vi "ILABW_RemoteCommandMgr.vi"(0 "action":string, 1 "data":string, 4 "errorIn":errorcluster) -> (5 "response":string, 7 "errorOut":string)   [LabVIEW 2012]
panel:
  in  "vi":string
  out "Control":bool
  out "Connection Status":string
  in  "Case Constant\n(See Context Help)":bool=TRUE
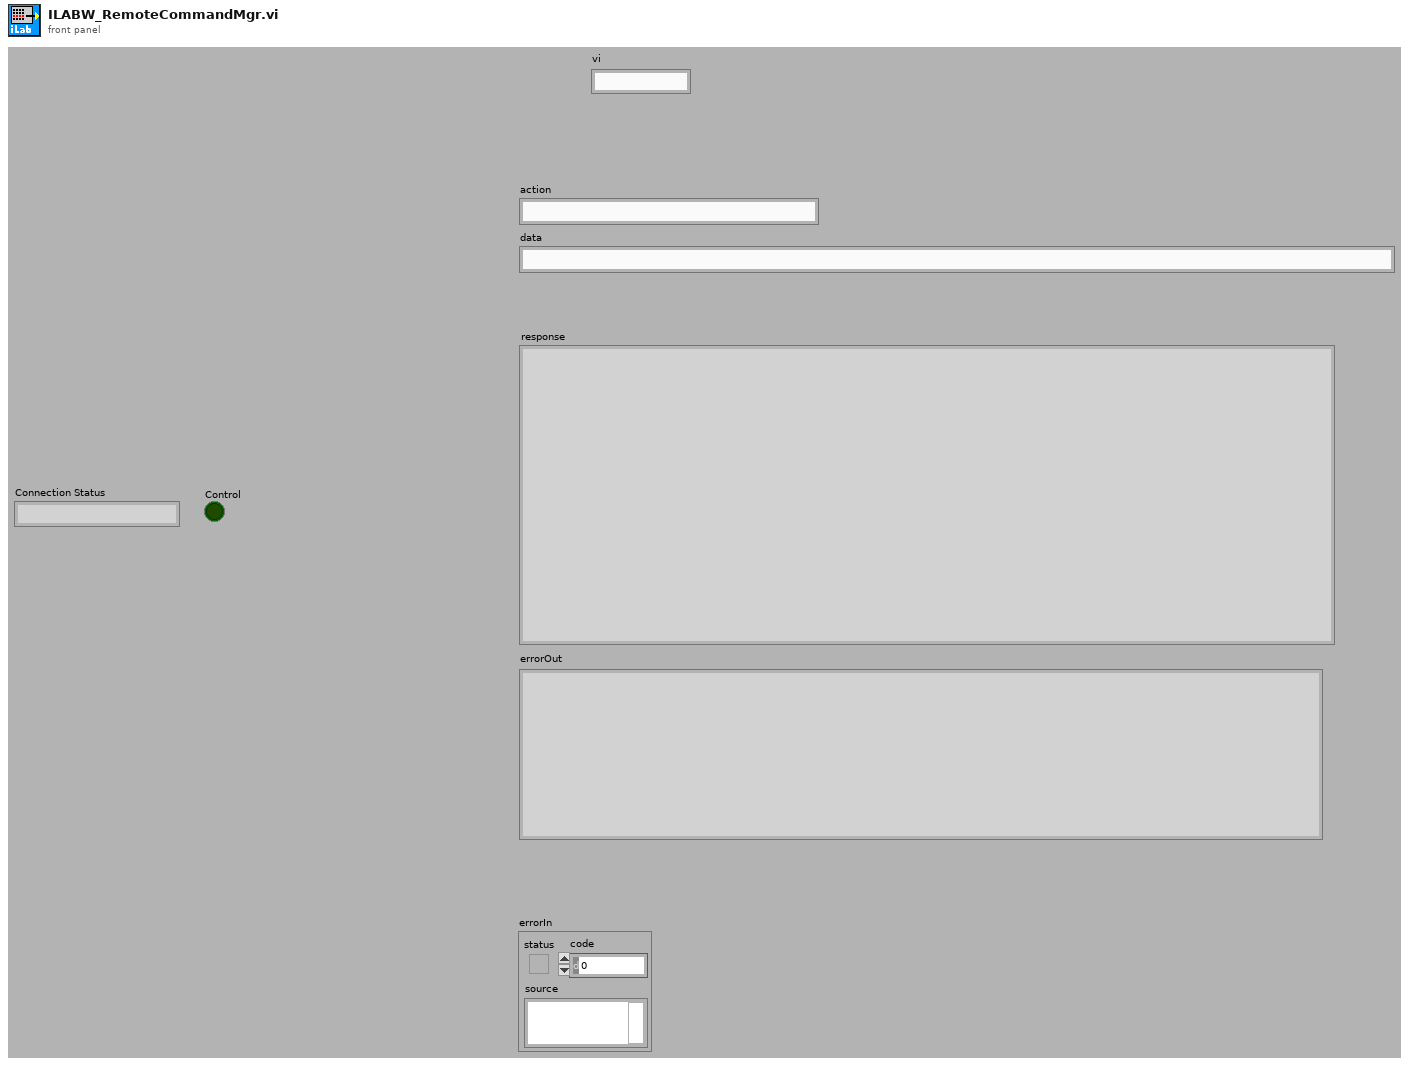
[diagram p1: front panel]
types:
  T1 = typedef "LVRemotePanelConnectionsTypeDef.ctl" = cluster{"VI Name":string, "Remote":string, "UserName":string, "Port":i32, "Status":enum32{"Viewing", "Waiting For Control", "Controlling"}, "Create Time":timestamp, "Status Time":timestamp, "Control End Time":timestamp}[]
  T2 = cluster{"VI Name":string, "Remote":string, "UserName":string, "Port":i32, "Status":enum32{"Viewing", "Waiting For Control", "Controlling"}, "Create Time":timestamp, "Status Time":timestamp, "Control End Time":timestamp}
  T3 = enum32{"Viewing", "Waiting For Control", "Controlling"}
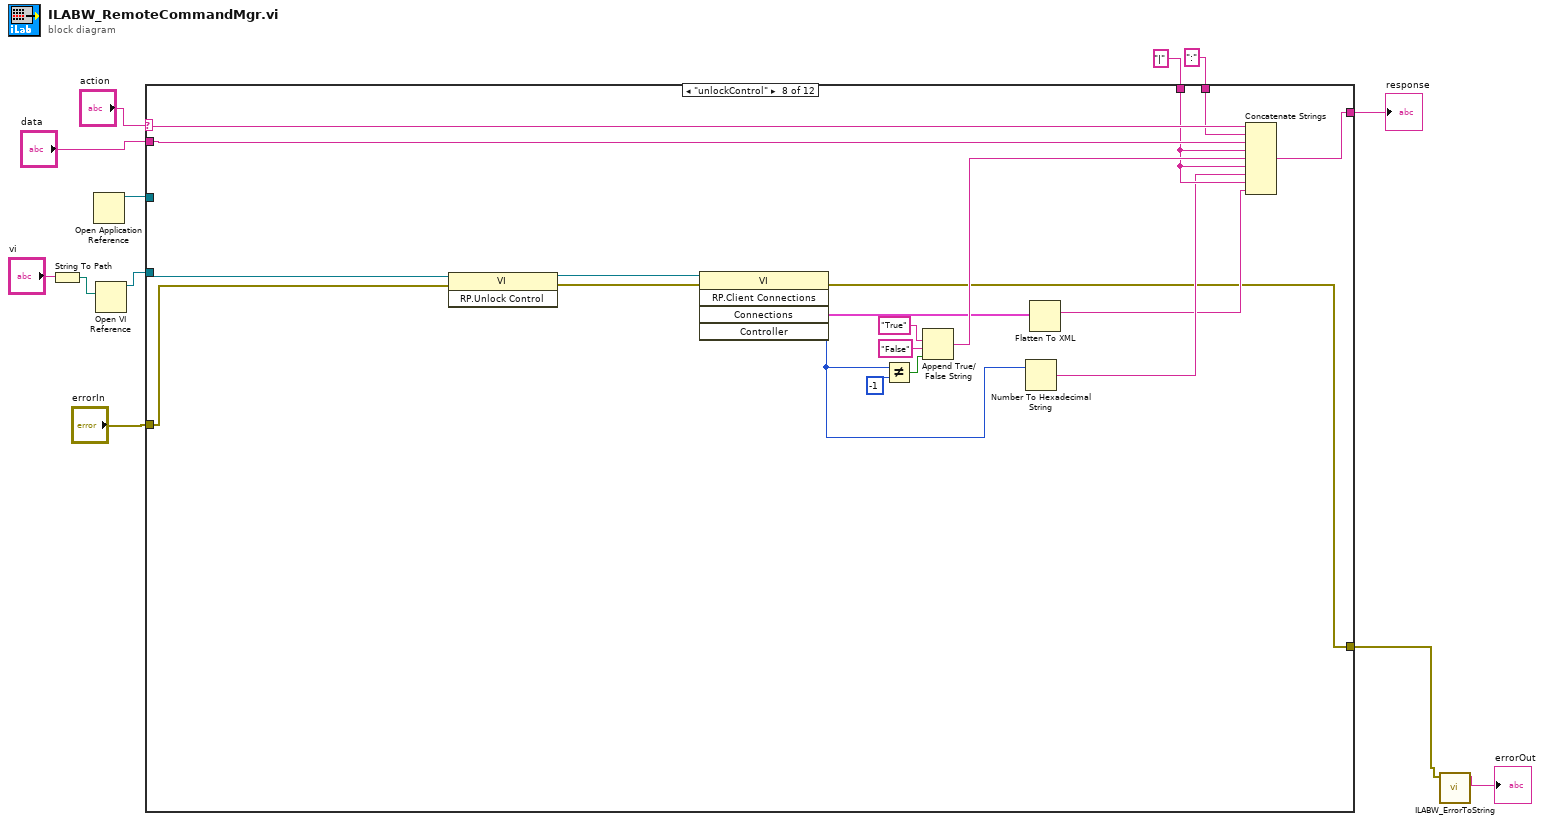
[diagram p0: block diagram]
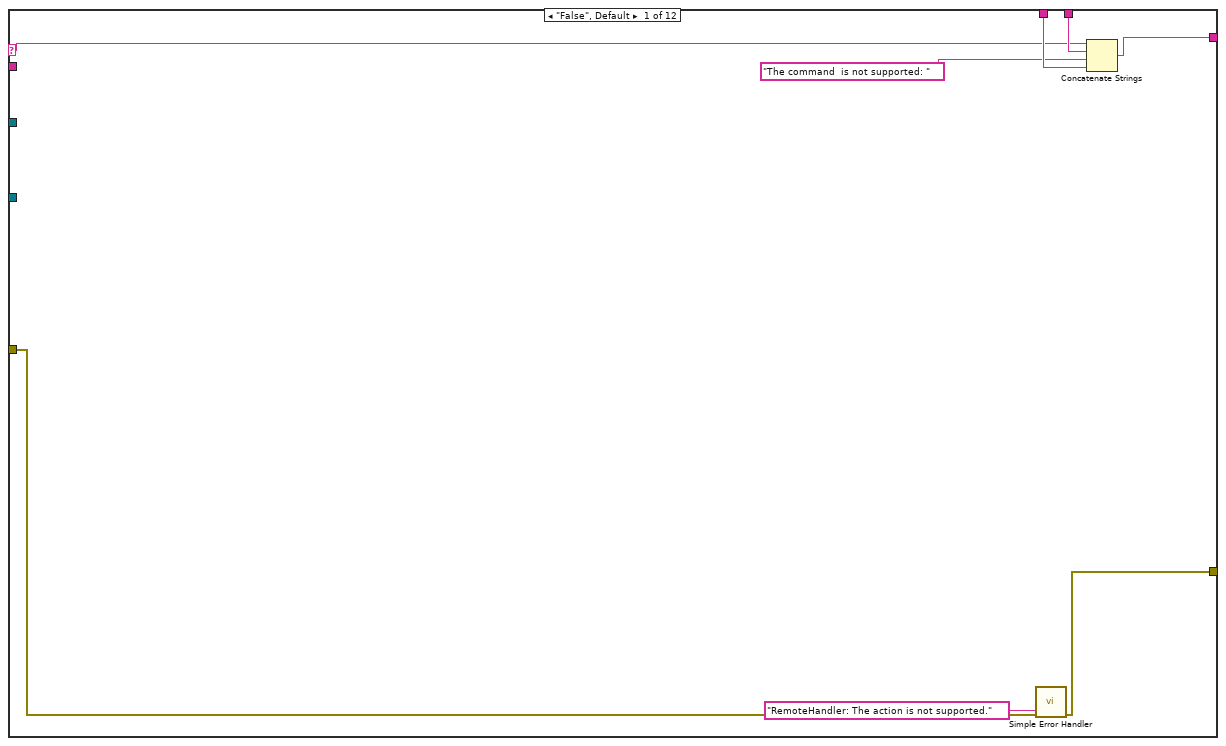
[diagram p2: hidden frame]
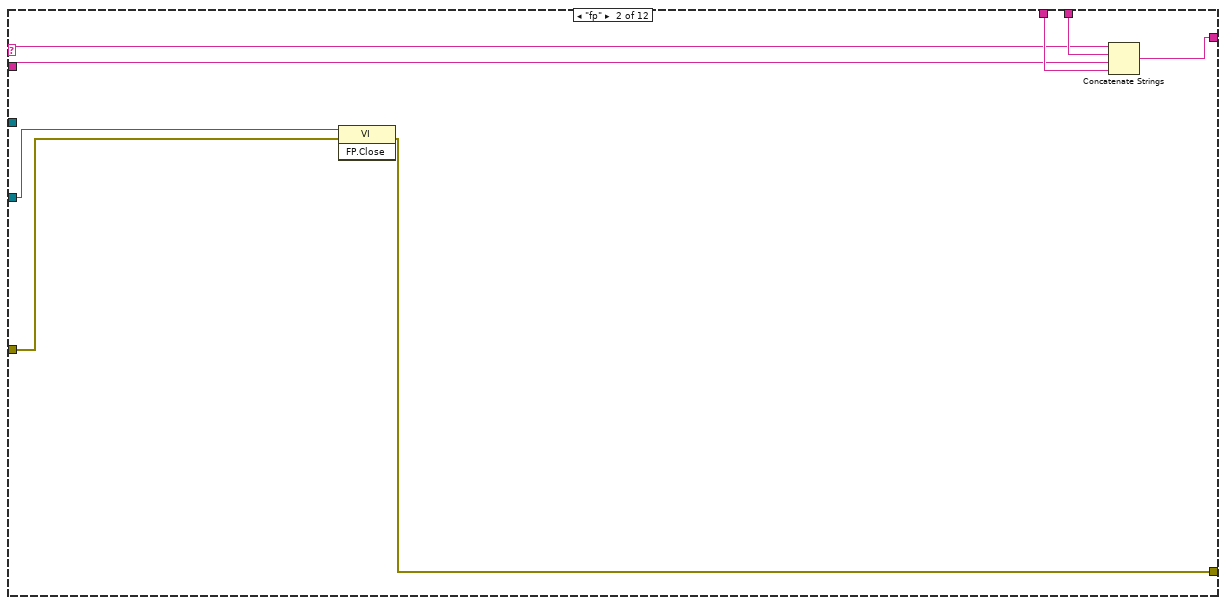
[diagram p3: hidden frame]
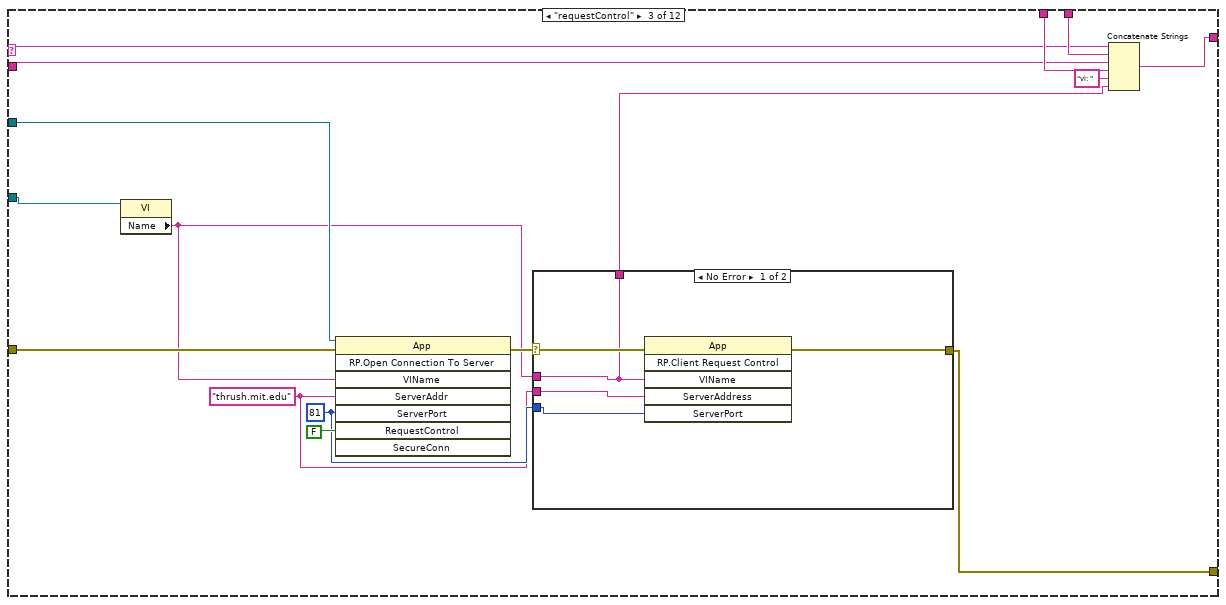
[diagram p4: hidden frame]
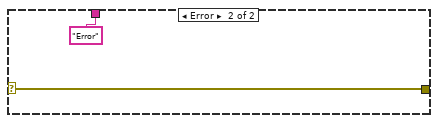
[diagram p5: hidden frame]
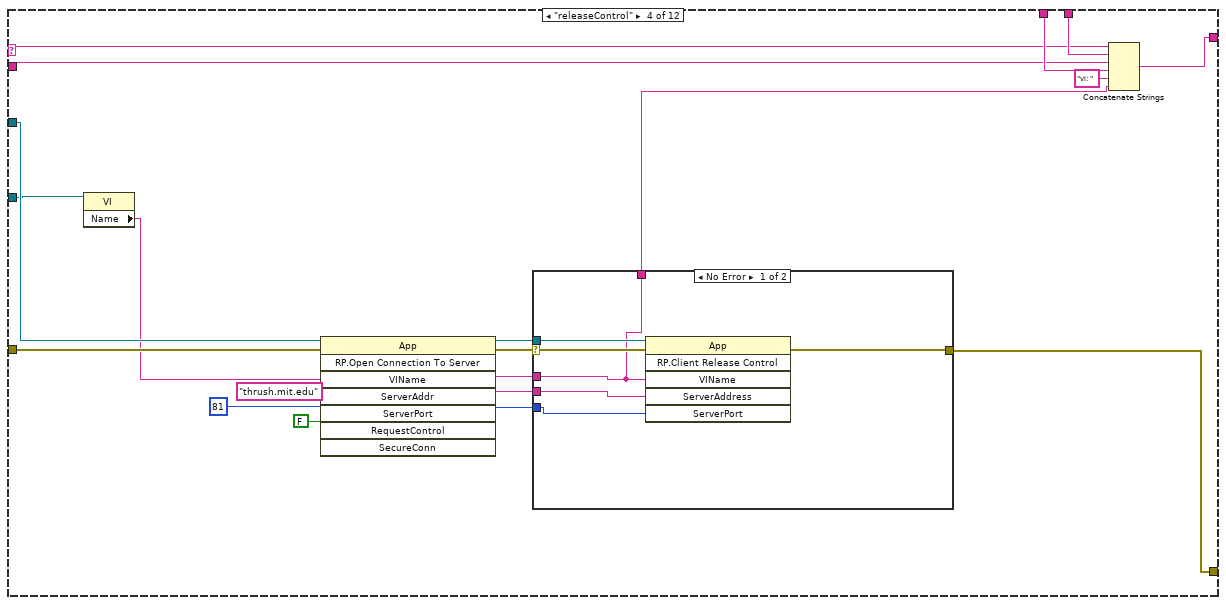
[diagram p6: hidden frame]
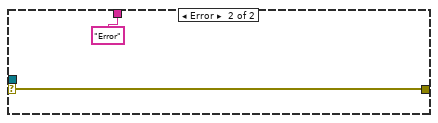
[diagram p7: hidden frame]
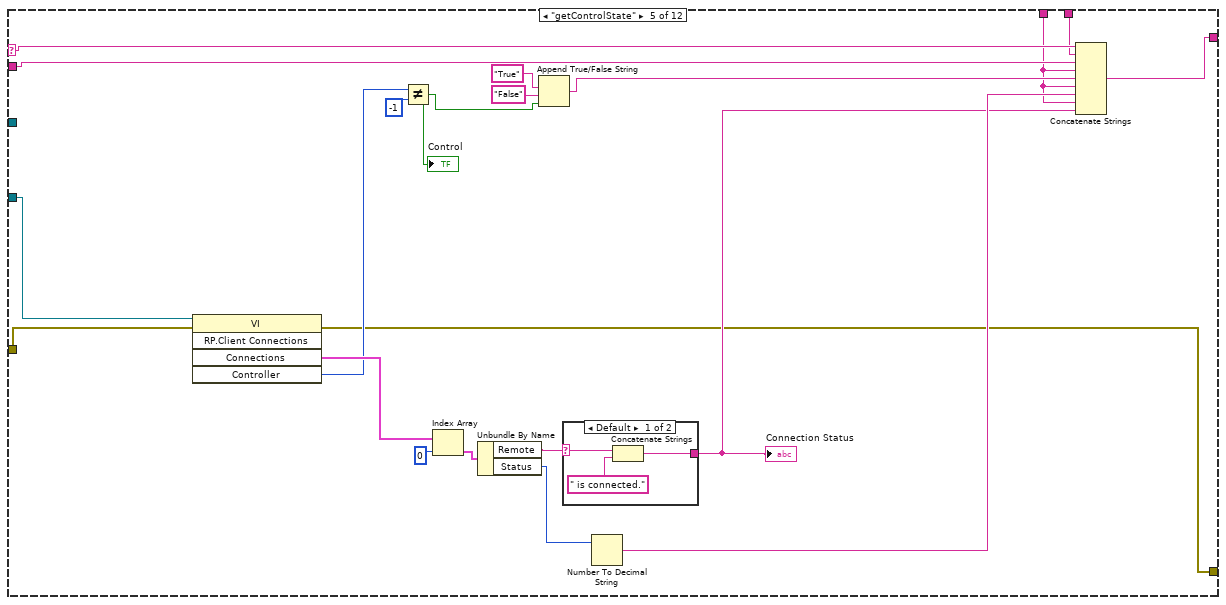
[diagram p8: hidden frame]
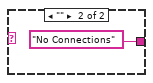
[diagram p9: hidden frame]
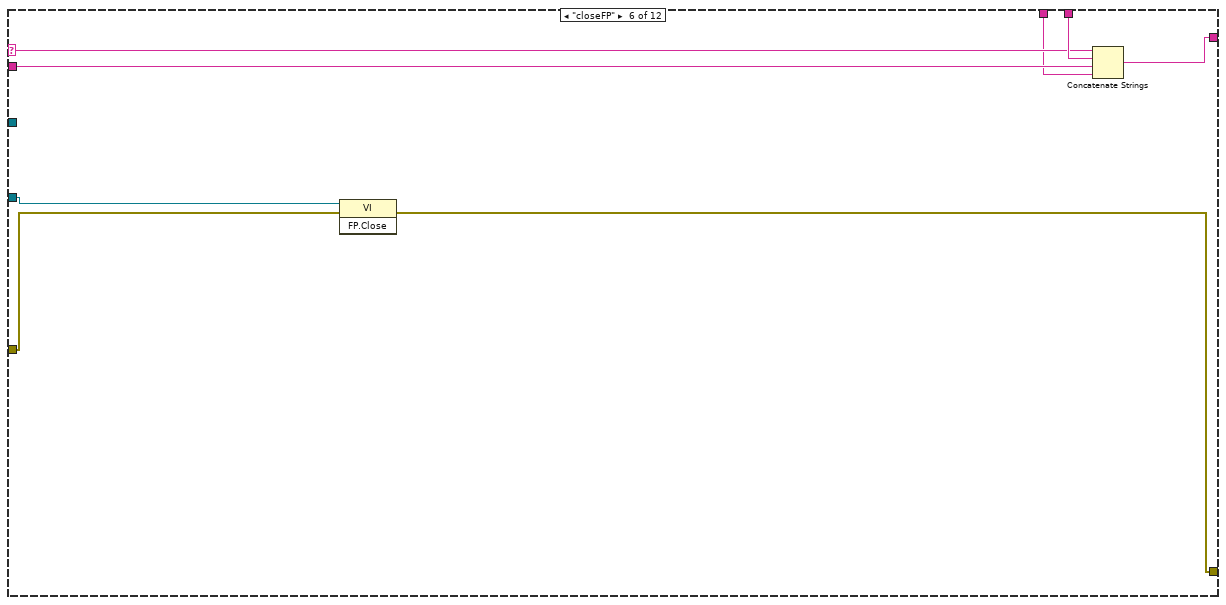
[diagram p10: hidden frame]
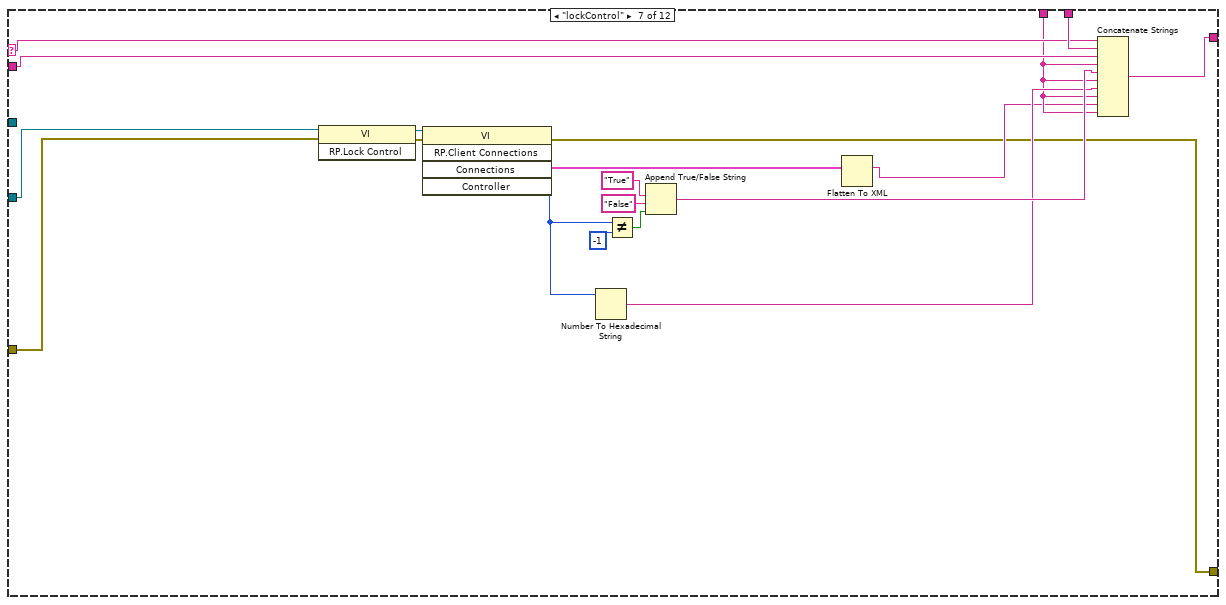
[diagram p11: hidden frame]
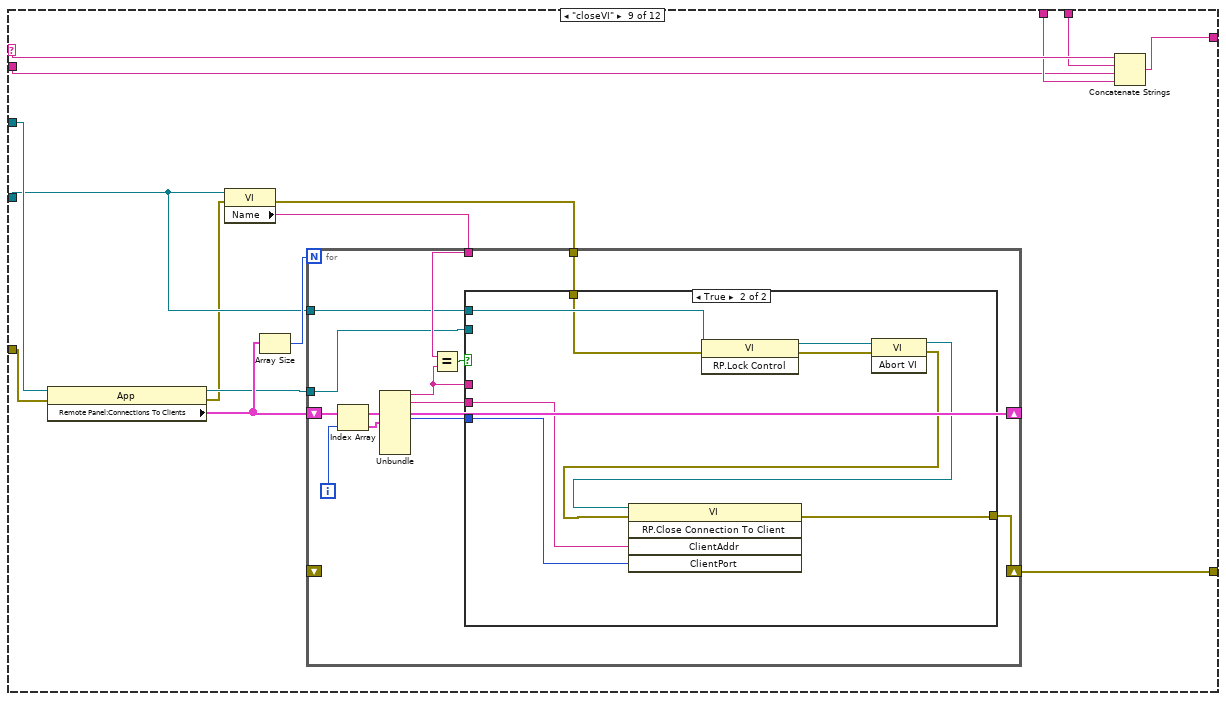
[diagram p12: hidden frame]
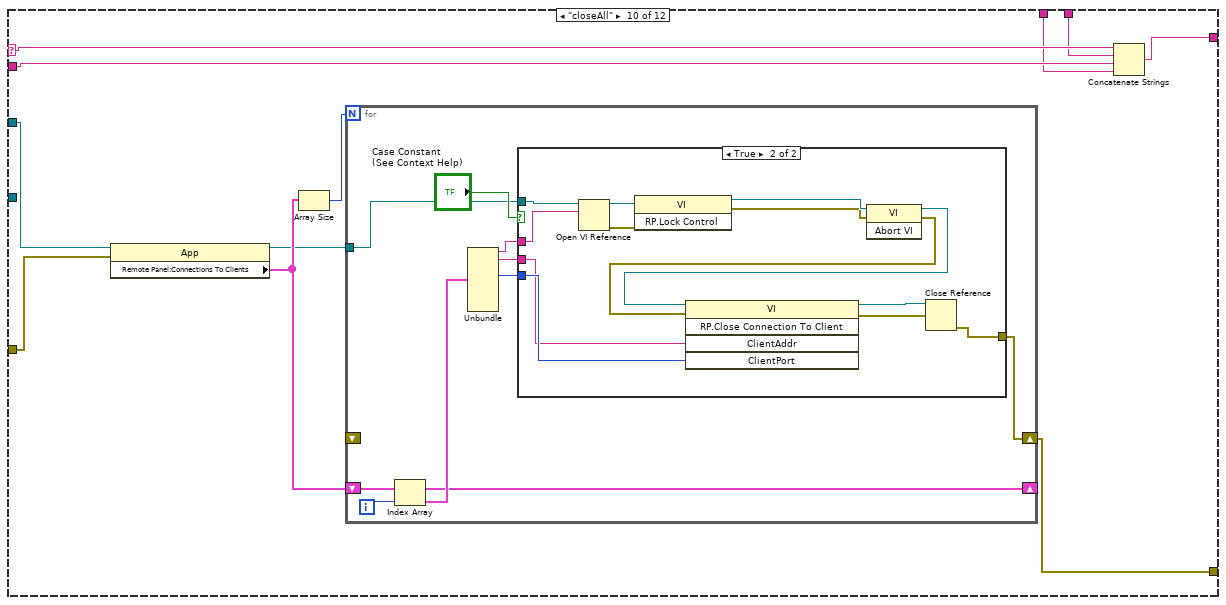
[diagram p14: hidden frame]
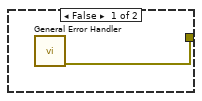
[diagram p15: hidden frame]
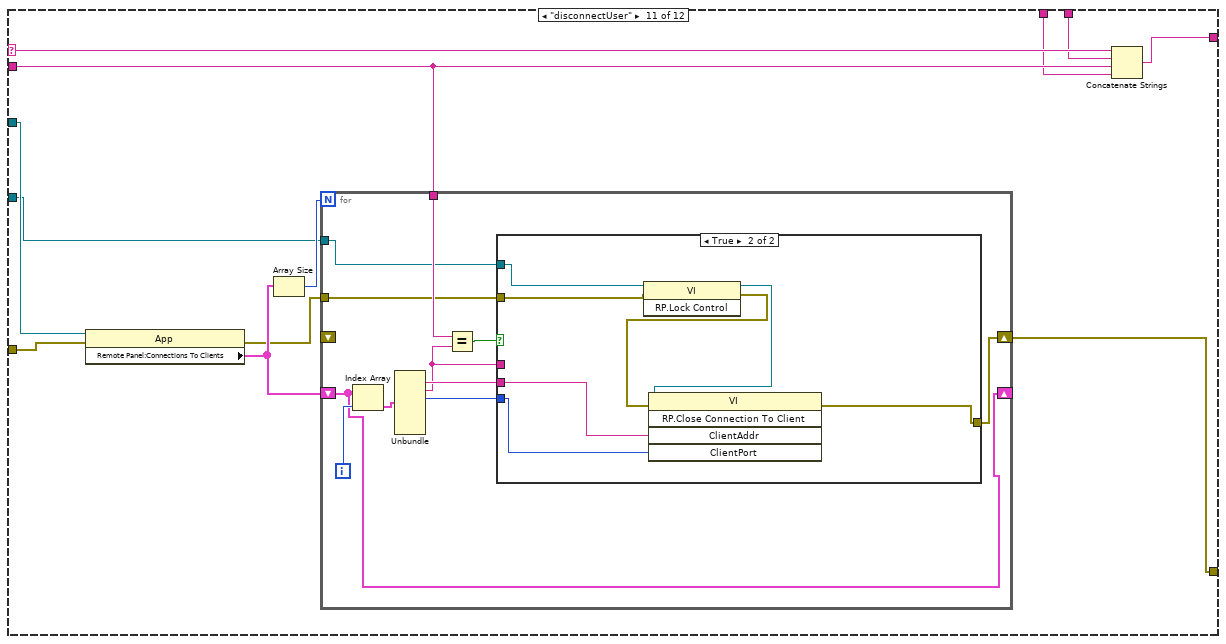
[diagram p16: hidden frame]
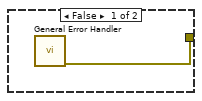
[diagram p17: hidden frame]
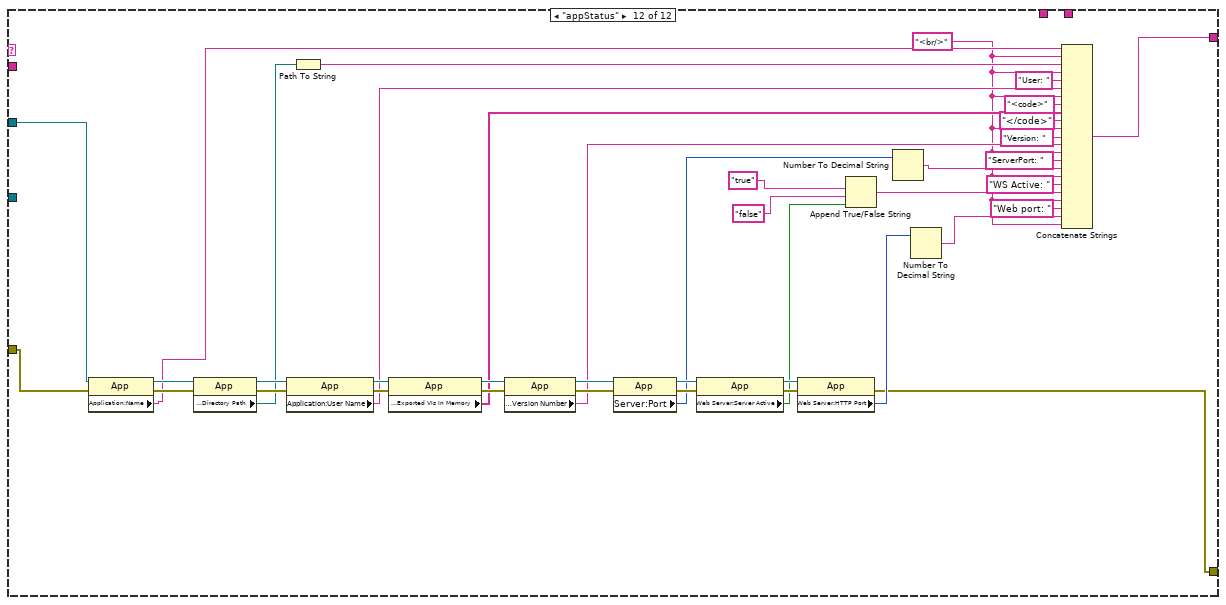
[diagram p18: hidden frame]
diagram:
  n1 = String To Path(string="vi") -> (path=w4:path)
  n2 = Open Application Reference() -> (3:w6:refnum<vi>)  [unwired: 4 in, 1 out]
  n3 = Open VI Reference(vi path=w4) -> (vi reference=w3:refnum<vi>)  [unwired: 5 in, 1 out]
  n4 = case shown="\"unlockControl\"" "action" {
    selector: "action" -> [w15 w25 w41 w65 w85 w107 w120 w140 w157 w190 w226 _]
    tunnel: "data" -> [_ w24 w34 w60 w84 w106 w119 w139 w153 w189 w225 _]
    tunnel: [w20 w28 w44 w68 w97 w109 w128 w147 w162 w193 w230 w252] -> w11
    tunnel: "errorIn" -> [w13 w21 w37 w59 w79 w103 w111 w130 w158 w192 w227 w289]
    tunnel: ":" -> [w18 w26 w42 w66 w81 w108 w121 w138 w156 w188 w224 _]
    tunnel: "|" -> [w17 w27 w43 w67 w80 w105 w115 w136 w155 w187 w223 _]
    tunnel: w6 -> [_ _ w36 w58 _ _ _ _ w154 w186 w222 w251]
    tunnel: w3 -> [_ w22 w35 w57 w78 w104 w112 w131 w151 _ w221 _]
    tunnel: [w14 w23 w32 w54 w77 w102 w110 w129 w148 w185 w219 w250] -> w2
    frame "False", Default {
      (unwired) "The" ("message")
      n5 = call <vilib>:"Simple Error Handler.vi"("error source (\" \")"="RemoteHandler: The action is not supported." ("error source (\" \")"), "error in (no error)"=w13) -> ("error out"=w14:errorcluster)  [unwired: 1 in, 6 out]
      n6 = Concatenate Strings(w15, w18, "The command  is not supported: " ("string"), w17) -> (w20:string)
    }
    frame "fp" {
      n7 = invoke class="VI" method="FP.Close"(reference=w22, error in=w21) -> (error out=w23:errorcluster)  [unwired: 1 in, 2 out]
      n8 = Concatenate Strings(w25, w26, w24, w27) -> (w28:string)
    }
    frame "requestControl" {
      w39 = 81 ("Server Port")
      w31 = "thrush.mit.edu" ("Server Address")
      n9 = property class="VI"(reference=w35) -> ("Name"=w33:string)  [unwired: 1 in, 2 out]
      n10 = invoke class="App" method="RP.Open Connection To Server"(reference=w36, error in=w37, "VIName"=w33, "ServerAddr"=w31, "ServerPort"=w39, "RequestControl"=FALSE ("Request Control")) -> (error out=w38:errorcluster)  [unwired: 2 in, 7 out]
      n11 = case shown="No Error" w38 {
        selector: w38 -> [w49 w51]
        tunnel: w33 -> [w45 _]
        tunnel: w31 -> [w48 _]
        tunnel: w39 -> [w47 _]
        tunnel: [w46 w51] -> w32
        tunnel: [w45 "Error" ("Name")] -> w29
        frame No Error {
          n12 = invoke class="App" method="RP.Client Request Control"(error in=w49, "VIName"=w45, "ServerAddress"=w48, "ServerPort"=w47) -> (error out=w46:errorcluster)  [unwired: 2 in, 5 out]
        }
        frame Error {
        }
      }
      n13 = Concatenate Strings(w41, w42, w34, w43, "vi: " ("string"), w29) -> (w44:string)
    }
    frame "releaseControl" {
      w62 = 81 ("Server Port")
      w63 = "thrush.mit.edu" ("Server Address")
      n14 = property class="VI"(reference=w57) -> ("Name"=w56:string)  [unwired: 1 in, 2 out]
      n15 = invoke class="App" method="RP.Open Connection To Server"(reference=w58, error in=w59, "VIName"=w56, "ServerAddr"=w63, "ServerPort"=w62, "RequestControl"=FALSE ("Request Control")) -> (reference out=w55:refnum<vi>, error out=w61:errorcluster)  [unwired: 2 in, 6 out]
      n16 = case shown="No Error" w61 {
        selector: w61 -> [w74 w76]
        tunnel: w56 -> [w69 _]
        tunnel: w63 -> [w73 _]
        tunnel: w62 -> [w72 _]
        tunnel: [w71 w76] -> w54
        tunnel: w55 -> [w70 _]
        tunnel: [w69 "Error" ("Name")] -> w53
        frame No Error {
          n17 = invoke class="App" method="RP.Client Release Control"(reference=w70, error in=w74, "VIName"=w69, "ServerAddress"=w73, "ServerPort"=w72) -> (error out=w71:errorcluster)  [unwired: 1 in, 5 out]
        }
        frame Error {
        }
      }
      n18 = Concatenate Strings(w65, w66, w60, w67, "vi: " ("string"), w53) -> (w68:string)
    }
    frame "getControlState" {
      n19 = invoke class="VI" method="RP.Client Connections"(reference=w78, error in=w79) -> (error out=w77:errorcluster, "Connections"=w96:T1, "Controller"=w93:i32)  [unwired: 3 in, 2 out]
      n20 = Not Equal?(x=w93, y=-1) -> (x != y?=w90:bool)
      "Control" <- w90
      n21 = Index Array(array=w96, index=0) -> (element=w91:T2)
      n22 = Unbundle By Name(w91) -> ("Remote"=w94:string, "Status"=w86:T3)
      n23 = Append True/False String(1:w90, 2:"False" ("false string"), 3:"True" ("true string")) -> (0:w87:string)  [unwired: 1 out]
      n24 = case shown="Default" w94 {
        selector: w94 -> [w100 _]
        tunnel: [w98 "No Connections"] -> w82
        frame Default {
          n25 = Concatenate Strings(w100, " is connected." ("string")) -> (w98:string)
        }
        frame "" {
        }
      }
      "Connection Status" <- w82
      n26 = Number To Decimal String(number=w86) -> (decimal integer string=w83:string)  [unwired: 1 out]
      n27 = Concatenate Strings(w85, w81, w84, w80, w87, w80, w83, w80, w82) -> (w97:string)
    }
    frame "closeFP" {
      n28 = invoke class="VI" method="FP.Close"(reference=w104, error in=w103) -> (error out=w102:errorcluster)  [unwired: 1 in, 2 out]
      n29 = Concatenate Strings(w107, w108, w106, w105) -> (w109:string)
    }
    frame "lockControl" {
      n30 = invoke class="VI" method="RP.Lock Control"(reference=w112, error in=w111) -> (reference out=w127:refnum<vi>, error out=w126:errorcluster)  [unwired: 1 in, 1 out]
      n31 = invoke class="VI" method="RP.Client Connections"(reference=w127, error in=w126) -> (error out=w110:errorcluster, "Connections"=w113:T1, "Controller"=w117:i32)  [unwired: 3 in, 2 out]
      n32 = Number To Hexadecimal String(2:w117) -> (0:w116:string)  [unwired: 1 out]
      n33 = Not Equal?(x=w117, y=-1) -> (x != y?=w124:bool)
      n34 = Append True/False String(1:w124, 2:"False" ("false string"), 3:"True" ("true string")) -> (0:w118:string)  [unwired: 1 out]
      n35 = Flatten To XML(anything=w113) -> (xml string=w114:string)
      n36 = Concatenate Strings(w120, w121, w119, w115, w118, w115, w116, w115, w114, w115) -> (w128:string)
    }
    frame "unlockControl" {
      n37 = invoke class="VI" method="RP.Unlock Control"(reference=w131, error in=w130) -> (reference out=w142:refnum<vi>, error out=w141:errorcluster)  [unwired: 1 in, 1 out]
      n38 = invoke class="VI" method="RP.Client Connections"(reference=w142, error in=w141) -> (error out=w129:errorcluster, "Connections"=w133:T1, "Controller"=w135:i32)  [unwired: 3 in, 2 out]
      n39 = Not Equal?(x=w135, y=-1) -> (x != y?=w145:bool)
      n40 = Append True/False String(1:w145, 2:"False" ("false string"), 3:"True" ("true string")) -> (0:w137:string)  [unwired: 1 out]
      n41 = Number To Hexadecimal String(2:w135) -> (0:w134:string)  [unwired: 1 out]
      n42 = Flatten To XML(anything=w133) -> (xml string=w132:string)
      n43 = Concatenate Strings(w140, w138, w139, w136, w137, w136, w134, w136, w132) -> (w147:string)
    }
    frame "closeVI" {
      n44 = property class="App"(reference=w154, error in=w158) -> (reference out=w159:refnum<vi>, error out=w150:errorcluster, "Remote Panel:Connections To Clients"=w160:T1)
      n45 = property class="VI"(reference=w151, error in=w150) -> (error out=w149:errorcluster, "Name"=w152:string)  [unwired: 1 out]
      n46 = Array Size(array=w160) -> (size(s)=w161:i32)
      n47 = for {
        N: w161 -> [_]
        shift-right: [w167] -> _
        shift-left: w160 -> [w167]
        tunnel: w152 -> [w172]
        shift-right: [w163] -> w148
        shift-left: _ -> [_]
        tunnel: w159 -> [w166]
        tunnel: w151 -> [w165]
        tunnel: w149 -> [w164]
        i -> [w174]
        n48 = Index Array(array=w167, index=w174) -> (element=w173:T2)
        n49 = Unbundle(w173) -> ("VI Name"=w168:string, "Remote"=w169:string, "Port"=w170:i32)  [unwired: 5 out]
        n50 = Equal?(x=w172, y=w168) -> (x = y?=w171:bool)
        n51 = case shown="True" w171 {
          tunnel: w170 -> [_ w184]
          tunnel: w169 -> [_ w183]
          tunnel: w168 -> [_ _]
          tunnel: w166 -> [_ _]
          tunnel: w165 -> [_ w178]
          tunnel: w164 -> [w175 w177]
          tunnel: [w175 w176] -> w163
          frame False {
          }
          frame True {
            n52 = invoke class="VI" method="RP.Lock Control"(reference=w178, error in=w177) -> (reference out=w182:refnum<vi>, error out=w181:errorcluster)  [unwired: 1 in, 1 out]
            n53 = invoke class="VI" method="Abort VI"(reference=w182, error in=w181) -> (reference out=w179:refnum<vi>, error out=w180:errorcluster)  [unwired: 1 in, 1 out]
            n54 = invoke class="VI" method="RP.Close Connection To Client"(reference=w179, error in=w180, "ClientAddr"=w183, "ClientPort"=w184) -> (error out=w176:errorcluster)  [unwired: 1 in, 4 out]
          }
        }
      }
      n55 = Concatenate Strings(w157, w156, w153, w155) -> (w162:string)
    }
    frame "closeAll" {
      n56 = property class="App"(reference=w186, error in=w192) -> (reference out=w191:refnum<vi>, "Remote Panel:Connections To Clients"=w194:T1)  [unwired: 1 out]
      n57 = Array Size(array=w194) -> (size(s)=w195:i32)
      n58 = for {
        N: w195 -> [_]
        shift-right: [w198] -> _
        shift-left: w194 -> [w198]
        shift-right: [w200] -> w185
        shift-left: _ -> [_]
        tunnel: w191 -> [w196]
        i -> [w204]
        n59 = Index Array(array=w198, index=w204) -> (element=w203:T2)
        n60 = Unbundle(w203) -> ("VI Name"=w199:string, "Remote"=w201:string, "Port"=w202:i32)  [unwired: 5 out]
        n61 = case shown="True" "Case Constant\n(See Context Help)" {
          tunnel: w202 -> [_ w218]
          tunnel: w201 -> [_ w217]
          tunnel: [w205 w216] -> w200
          tunnel: w199 -> [_ w215]
          tunnel: w196 -> [_ w206]
          frame False {
            n62 = call <vilib>:"General Error Handler.vi"() -> ("error out"=w205:errorcluster)  [unwired: 2 in, 13 out]
          }
          frame True {
            n63 = Open VI Reference(application reference (local)=w206, vi path=w215) -> (vi reference=w210:refnum<vi>, error out=w209:errorcluster)  [unwired: 1 in, 3 out]
            n64 = invoke class="VI" method="RP.Lock Control"(reference=w210, error in=w209) -> (reference out=w208:refnum<vi>, error out=w207:errorcluster)  [unwired: 1 in, 1 out]
            n65 = invoke class="VI" method="Abort VI"(reference=w208, error in=w207) -> (reference out=w211:refnum<vi>, error out=w212:errorcluster)  [unwired: 1 in, 1 out]
            n66 = invoke class="VI" method="RP.Close Connection To Client"(reference=w211, error in=w212, "ClientAddr"=w217, "ClientPort"=w218) -> (reference out=w214:refnum<vi>, error out=w213:errorcluster)  [unwired: 1 in, 3 out]
            n67 = Close Reference(reference=w214, error in (no error)=w213) -> (error out=w216:errorcluster)
          }
        }
      }
      n68 = Concatenate Strings(w190, w188, w189, w187) -> (w193:string)
    }
    frame "disconnectUser" {
      n69 = property class="App"(reference=w222, error in=w227) -> (error out=w220:errorcluster, "Remote Panel:Connections To Clients"=w228:T1)  [unwired: 1 out]
      n70 = Array Size(array=w228) -> (size(s)=w229:i32)
      n71 = for {
        N: w229 -> [_]
        shift-right: [w235] -> _
        shift-left: w228 -> [w235]
        tunnel: w225 -> [w234]
        shift-right: [w236] -> w219
        shift-left: _ -> [_]
        tunnel: w221 -> [w233]
        tunnel: w220 -> [w232]
        i -> [w241]
        n72 = Index Array(array=w235, index=w241) -> (element=w240:T2)
        n73 = Unbundle(w240) -> ("Remote"=w237:string, "UserName"=w231:string, "Port"=w238:i32)  [unwired: 5 out]
        n74 = Equal?(x=w234, y=w231) -> (x = y?=w239:bool)
        n75 = case shown="True" w239 {
          tunnel: w238 -> [_ w249]
          tunnel: w237 -> [_ w248]
          tunnel: [w242 w244] -> w236
          tunnel: w231 -> [_ _]
          tunnel: w233 -> [_ w245]
          tunnel: w232 -> [_ w243]
          frame False {
            n76 = call <vilib>:"General Error Handler.vi"() -> ("error out"=w242:errorcluster)  [unwired: 2 in, 13 out]
          }
          frame True {
            n77 = invoke class="VI" method="RP.Lock Control"(reference=w245, error in=w243) -> (reference out=w247:refnum<vi>, error out=w246:errorcluster)  [unwired: 1 in, 1 out]
            n78 = invoke class="VI" method="RP.Close Connection To Client"(reference=w247, error in=w246, "ClientAddr"=w248, "ClientPort"=w249) -> (error out=w244:errorcluster)  [unwired: 1 in, 4 out]
          }
        }
      }
      n79 = Concatenate Strings(w226, w224, w225, w223) -> (w230:string)
    }
    frame "appStatus" {
      w253 = "<br/>" ("string")
      n80 = property class="App"(reference=w251, error in=w289) -> (reference out=w288:refnum<vi>, error out=w283:errorcluster, "Application:Name"=w274:string)
      n81 = property class="App"(reference=w288, error in=w283) -> (reference out=w287:refnum<vi>, error out=w282:errorcluster, "Application:Directory Path"=w272:path)
      n82 = property class="App"(reference=w287, error in=w282) -> (reference out=w286:refnum<vi>, error out=w281:errorcluster, "Application:User Name"=w270:string)
      n83 = Path To String(path=w272) -> (string=w273:string)
      n84 = property class="App"(reference=w286, error in=w281) -> (reference out=w285:refnum<vi>, error out=w280:errorcluster, "Application:Exported VIs In Memory"=w268:string[])
      n85 = property class="App"(reference=w285, error in=w280) -> (reference out=w284:refnum<vi>, error out=w279:errorcluster, "Application:Version Number"=w265:string)
      n86 = property class="App"(reference=w284, error in=w279) -> (reference out=w275:refnum<vi>, error out=w276:errorcluster, "Server:Port"=w262:u32)
      n87 = property class="App"(reference=w275, error in=w276) -> (reference out=w278:refnum<vi>, error out=w277:errorcluster, "Web Server:Server Active"=w260:bool)
      n88 = property class="App"(reference=w278, error in=w277) -> (error out=w250:errorcluster, "Web Server:HTTP Port"=w255:u16)  [unwired: 1 out]
      n89 = Append True/False String(1:w260, 2:"false" ("false string"), 3:"true" ("true string")) -> (0:w259:string)  [unwired: 1 out]
      n90 = Number To Decimal String(number=w262) -> (decimal integer string=w263:string)  [unwired: 1 out]
      n91 = Number To Decimal String(number=w255) -> (decimal integer string=w254:string)  [unwired: 1 out]
      n92 = Concatenate Strings(w274, w253, w273, w253, "User: " ("string"), w270, w253, "<code>" ("string"), w268, "</code>" ("string"), w253, "Version: " ("string"), w265, w253, "ServerPort: " ("string"), w263, w253, "WS Active: " ("string"), w259, w253, "Web port: " ("string"), w254, w253) -> (w252:string)
    }
  }
  "response" <- w11
  n93 = call "ILABW_ErrorToString.vi"("errorIn"=w2) -> ("errorOut"=→"errorOut":string)  [unwired: 10 in]
